vi "MSScript_SubVI_ArrayGetIndice.vi"(3 "indice string in":string) -> (0 "error":bool, 1 "x:y":i32[](array[numeric]))   [LabVIEW 2018, in "MSScript.lvclass"]
uses:
  MSScript.lvclass
  MSScript_Transform_Extended.vi
  MSScript_Transform_UIntArray.vi
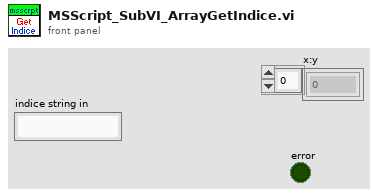
[diagram p1: front panel]
types:
  T1 = enum16{"Scalar", "ScalarArray", "Var", "VarArray", "Error"}
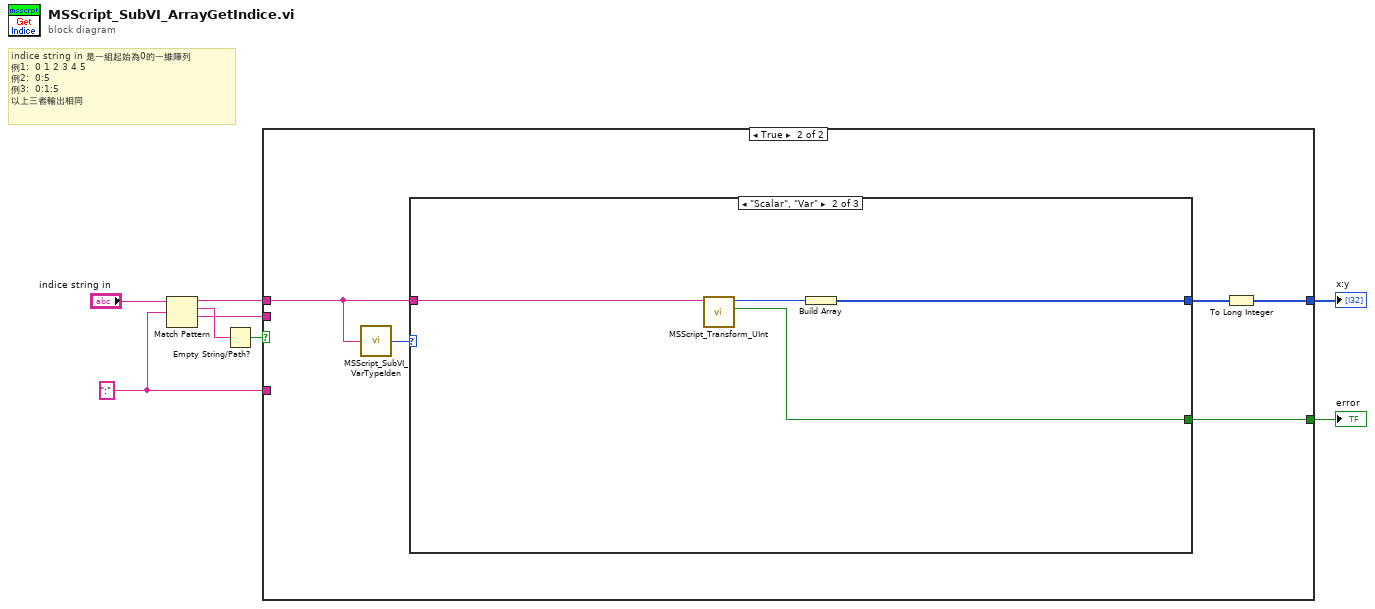
[diagram p0: block diagram]
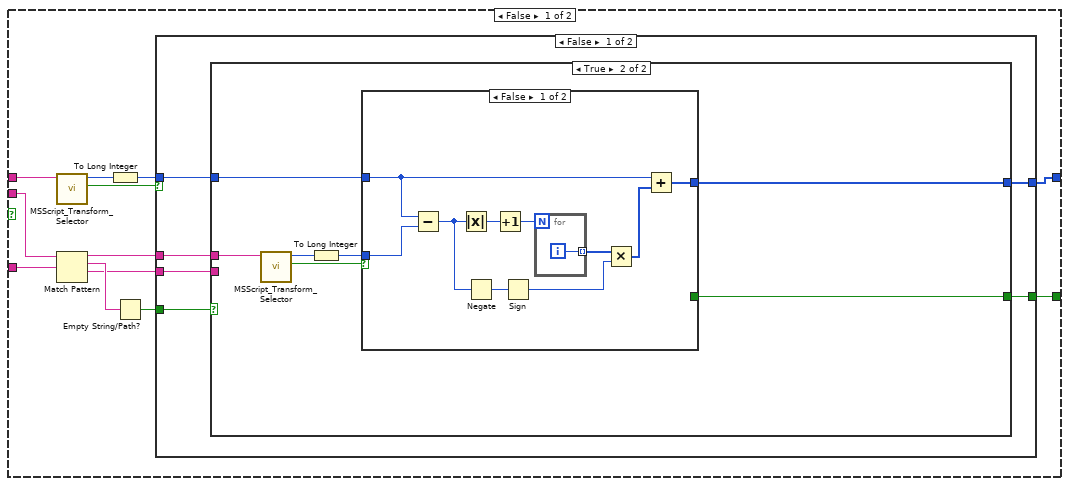
[diagram p2: hidden frame]
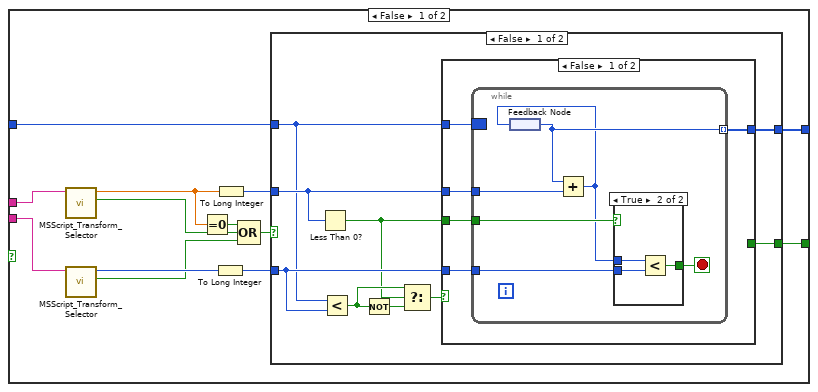
[diagram p3: hidden frame]
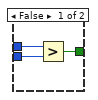
[diagram p4: hidden frame]
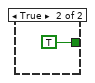
[diagram p5: hidden frame]
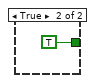
[diagram p6: hidden frame]
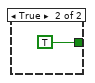
[diagram p7: hidden frame]
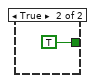
[diagram p8: hidden frame]
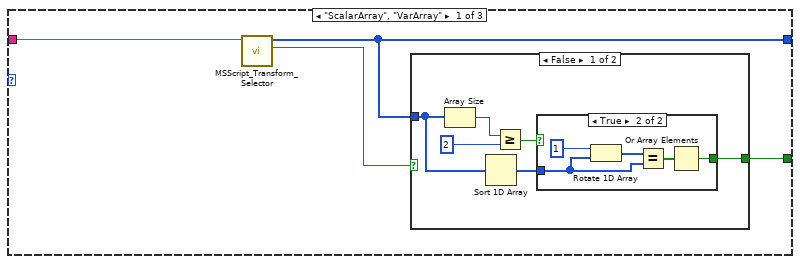
[diagram p9: hidden frame]
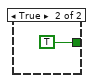
[diagram p11: hidden frame]
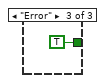
[diagram p12: hidden frame]
diagram:
  w1 = ":" ("regular expression")
  # "indice string in 是一組起始為0的一維陣列\n例1:  0 1 2 3 4 5\n例2:  0:5\n例3:  0:1:5\n以上三者輸出相同"
  n1 = Match Pattern(string="indice string in", regular expression=w1) -> (before substring=w4:string, match substring=w7:string, after substring=w3:string)  [unwired: 1 in, 1 out]
  n2 = Empty String/Path?(string/path=w7) -> (empty?=w5:bool)
  n3 = case shown="True" w5 {
    tunnel: [w20 w88] -> w6
    tunnel: w4 -> [w12 w91]
    tunnel: w3 -> [w18 _]
    tunnel: [w19 w92] -> w2
    tunnel: w1 -> [w17 _]
    frame False {
      n4 = call-poly "MSScript_Transform_Selector.vi"("string in"=w12) -> ("Value Error?"=w9:bool, "Value Output"=w11:u64)  [unwired: 8 in, 1 out]
      n5 = Match Pattern(string=w18, regular expression=w17) -> (before substring=w14:string, match substring=w16:string, after substring=w13:string)  [unwired: 1 in, 1 out]
      n6 = To Long Integer(number=w11) -> (32bit integer=w10:i32)
      n7 = Empty String/Path?(string/path=w16) -> (empty?=w15:bool)
      n8 = case shown="False" w9 {
        tunnel: [w23 _] -> w20
        tunnel: [w22 TRUE] -> w19
        tunnel: w15 -> [w26 _]
        tunnel: w14 -> [w25 _]
        tunnel: w13 -> [w24 _]
        tunnel: w10 -> [w21 _]
        frame False {
          n9 = case shown="True" w26 {
            tunnel: w21 -> [w38 w74]
            tunnel: w25 -> [w31 w70]
            tunnel: w24 -> [w32 _]
            tunnel: [w34 w73] -> w23
            tunnel: [w33 w71] -> w22
            frame False {
              n10 = call-poly "MSScript_Transform_Selector.vi"("Check_Str"=w31) -> ("Value Error?"=w29:bool, "Value Output"=w30:ext)  [unwired: 8 in, 1 out]
              n11 = call-poly "MSScript_Transform_Selector.vi"("string in"=w32) -> ("Value Error?"=w27:bool, "Value Output"=w28:u64)  [unwired: 8 in, 1 out]
              n12 = Equal To 0?(x=w30) -> (x = 0?=w37:bool)
              n13 = To Long Integer(number=w28) -> (32bit integer=w35:i32)
              n14 = To Long Integer(number=w30) -> (32bit integer=w36:i32)
              n15 = Compound Arithmetic op=OR(w37, w29, w27) -> (w39:bool)
              n16 = case shown="False" w39 {
                tunnel: w38 -> [w43 _]
                tunnel: w36 -> [w44 _]
                tunnel: w35 -> [w45 _]
                tunnel: [w41 _] -> w34
                tunnel: [w40 TRUE] -> w33
                frame False {
                  n17 = Less Than 0?(x=w44) -> (x < 0?=w42:bool)
                  n18 = Less?(x=w43, y=w45) -> (x < y?=w48:bool)
                  n19 = Not(x=w48) -> (.not. x?=w47:bool)
                  n20 = Select(t=w48, s=w42, f=w47) -> (s? t:f=w46:bool)
                  n21 = case shown="False" w46 {
                    tunnel: w45 -> [w52 _]
                    tunnel: w44 -> [w53 _]
                    tunnel: w43 -> [w50 _]
                    tunnel: w42 -> [w51 _]
                    tunnel: [w49 _] -> w41
                    tunnel: [_ TRUE] -> w40
                    frame False {
                      n22 = while {
                        tunnel: w53 -> [w59]
                        tunnel: w52 -> [w55]
                        tunnel: w51 -> [w57]
                        border: w50 -> [_]
                        tunnel: [w58] -> w49 mode=indexing
                        stop <- w54 stop-if-true
                        n23 = feedback #1() -> (w58:i32)
                        n24 = Add(x=w58, y=w59) -> (x+y=w56:i32)
                        n25 = feedback-in #1(w56) -> ()
                        n26 = case shown="True" w57 {
                          tunnel: w56 -> [w62 w65]
                          tunnel: w55 -> [w61 w64]
                          tunnel: [w60 w63] -> w54
                          frame False {
                            n27 = Greater?(x=w62, y=w61) -> (0:w60:bool)
                          }
                          frame True {
                            n28 = Less?(x=w65, y=w64) -> (x < y?=w63:bool)
                          }
                        }
                      }
                    }
                    frame True {
                    }
                  }
                }
                frame True {
                }
              }
            }
            frame True {
              n29 = call-poly "MSScript_Transform_Selector.vi"("string in"=w70) -> ("Value Error?"=w69:bool, "Value Output"=w68:u64)  [unwired: 8 in, 1 out]
              n30 = To Long Integer(number=w68) -> (32bit integer=w72:i32)
              n31 = case shown="False" w69 {
                tunnel: w74 -> [w77 _]
                tunnel: [w76 _] -> w73
                tunnel: w72 -> [w75 _]
                tunnel: [_ TRUE] -> w71
                frame False {
                  n32 = Subtract(x=w77, y=w75) -> (x-y=w81:i32)
                  n33 = Absolute Value(x=w81) -> (abs(x)=w78:i32)
                  n34 = Negate(x=w81) -> (-x=w80:i32)
                  n35 = Increment(x=w78) -> (x+1=w79:i32)
                  n36 = Sign(1:w80) -> (0:w84:i32)
                  n37 = for {
                    N: w79 -> [_]
                    tunnel: [w85] -> w83 mode=indexing
                    i -> [w85]
                  }
                  n38 = Multiply(x=w83, y=w84) -> (x*y=w82:i32[])
                  n39 = Add(x=w77, y=w82) -> (x+y=w76:i32[])
                }
                frame True {
                }
              }
            }
          }
        }
        frame True {
        }
      }
    }
    frame True {
      n40 = call "MSScript_SubVI_VarTypeIden.vi"("Var in"=w91) -> ("Type"=w90:T1)
      n41 = case shown="\"Scalar\", \"Var\"" w90 {
        tunnel: [w96 w109 TRUE ("Value Error?")] -> w92
        tunnel: [w95 w110 _] -> w89
        tunnel: w91 -> [w93 w112 _]
        frame "ScalarArray", "VarArray" {
          n42 = call-poly "MSScript_Transform_Selector.vi"("Check_Str"=w93) -> ("Value Error?"=w94:bool, "Value Output"=w95:u64[])  [unwired: 8 in, 1 out]
          n43 = case shown="False" w94 {
            tunnel: w95 -> [w98 _]
            tunnel: [w102 TRUE] -> w96
            frame False {
              n44 = Array Size(array=w98) -> (size(s)=w97:i32)
              n45 = Sort 1D Array(array=w98) -> (sorted array=w101:u64[])
              n46 = Greater Or Equal?(x=w97, y=2 ("n")) -> (x >= y?=w99:bool)
              n47 = case shown="True" w99 {
                tunnel: [_ w105] -> w102
                tunnel: w101 -> [_ w103]
                frame False {
                }
                frame True {
                  n48 = Rotate 1D Array(1:w103, 2:1 ("n")) -> (0:w104:u64[])
                  n49 = Equal?(x=w104, y=w103) -> (x = y?=w106:bool[])
                  n50 = Or Array Elements(Boolean array=w106) -> (logical OR=w105:bool)
                }
              }
            }
            frame True {
            }
          }
        }
        frame "Scalar", "Var" {
          n51 = call "MSScript_Transform_UInt.vi"("string in"=w112) -> ("Value Error?"=w109:bool, "Value Output"=w111:u64)  [unwired: 8 in, 1 out]
          n52 = Build Array(w111) -> (w110:u64[])
        }
        frame "Error" {
        }
      }
      n53 = To Long Integer(number=w89) -> (32bit integer=w88:i32[])
    }
  }
  "x:y" <- w6
  "error" <- w2
